vi "Load Config.vi"(8 "error in (no error)":errorcluster, 11 "StrainChannel in":refnum<class "StrainChannel.lvclass">) -> (0 "error out":errorcluster, 3 "StrainChannel out":refnum<class "StrainChannel.lvclass">)   [LabVIEW 2023, in "VolatusDAQConfig.lvlib" / "StrainChannel.lvclass"]
uses:
  StrainChannel.lvclass
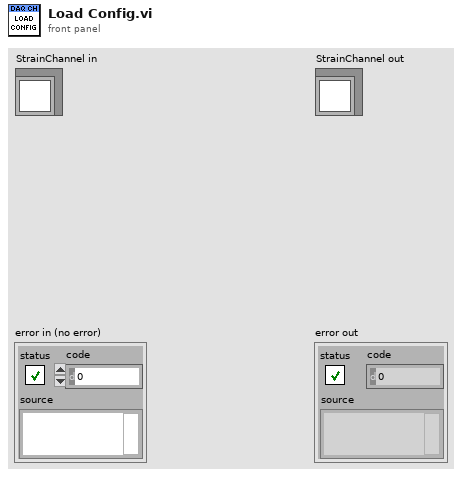
[diagram p1: front panel]
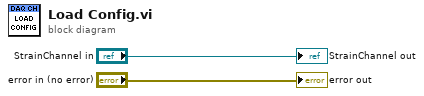
[diagram p0: block diagram]
diagram:
  "error out" <- "error in (no error)"
  "StrainChannel out" <- "StrainChannel in"
